vi "5p1_HW_Task2_UCweesesr.vi"() -> ()   [LabVIEW 2016]
panel:
  out "Result":string
  in  "Derivative of x":dbl
  in  "Second Derivative of x":dbl
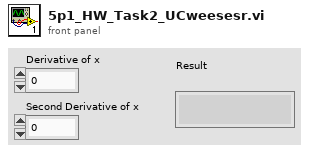
[diagram p1: front panel]
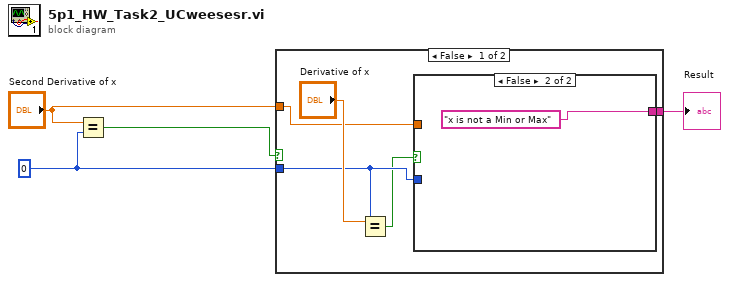
[diagram p0: block diagram]
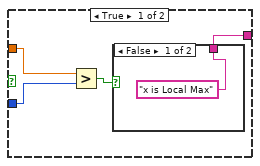
[diagram p2: hidden frame]
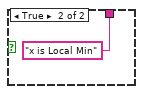
[diagram p3: hidden frame]
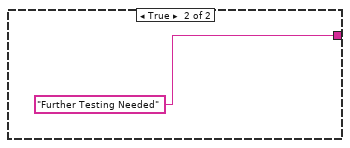
[diagram p4: hidden frame]
diagram:
  w1 = 0
  n1 = Equal?(x="Second Derivative of x", y=w1) -> (x = y?=w4:bool)
  n2 = case shown="False" w4 {
    tunnel: [w6 "Further Testing Needed"] -> w3
    tunnel: "Second Derivative of x" -> [w8 _]
    tunnel: w1 -> [w7 _]
    frame False {
      n3 = Equal?(x="Derivative of x", y=w7) -> (x = y?=w5:bool)
      n4 = case shown="False" w5 {
        tunnel: w8 -> [w12 _]
        tunnel: w7 -> [w11 _]
        tunnel: [w10 "x is not a Min or Max"] -> w6
        frame True {
          n5 = Greater?(x=w12, y=w11) -> (0:w13:bool)
          n6 = case shown="False" w13 {
            tunnel: ["x is Local Max" "x is Local Min"] -> w10
            frame False {
            }
            frame True {
            }
          }
        }
        frame False {
        }
      }
    }
    frame True {
    }
  }
  "Result" <- w3
